vi "Write Test Execs.vi"(10 "Test Execs":refnum<data-value>[](array[refnum]), 11 "Parallel in":refnum<class "Parallel.lvclass">) -> (3 "Parallel out":refnum<class "Parallel.lvclass">)   [LabVIEW 2017, in "Test Executive.lvlib" / "Parallel.lvclass"]
uses:
  <vilib>/gpm_packages/@cs/test-executive/Source/Test Executive/Parallel/Parallel.lvclass
  <vilib>/gpm_packages/@cs/test-executive/Source/Test Executive/ITestExecutive/ITest Executive.lvclass
  <vilib>/gpm_packages/@cs/test-executive/Source/Test Executive/Parallel/Parallel.lvclass/Parallel.ctl
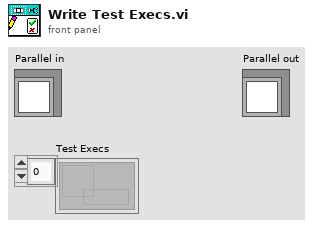
[diagram p1: front panel]
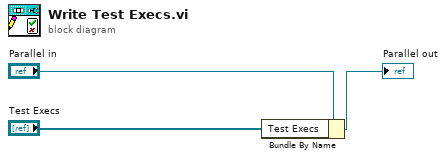
[diagram p0: block diagram]
diagram:
  n1 = Bundle By Name(cluster="Parallel in", "Test Execs"="Test Execs") -> (→"Parallel out":refnum<class "Parallel.lvclass">)
